vi "Send Command.vi"(7 "VolatusAPI":refnum<class "VolatusAPI.lvclass">, 8 "error in (no error)":errorcluster, 10 "Value":bool, 11 "2WayValve in":refnum<class "2WayValveH.lvclass">) -> (0 "error out":errorcluster, 3 "2WayValve out":refnum<class "2WayValveH.lvclass">)   [LabVIEW 2020, in "VolatusGUIElements.lvlib" / "2WayValveH.lvclass"]
uses:
  2WayValveH.lvclass
  Volatus/VolatusAPI/VolatusAPI.lvclass
  2WayValveH.lvclass/2WayValveH.ctl
  messages/CmdDigital/Class/Msg.lvclass/Msg.ctl
  Volatus/VolatusAPI/VolatusAPI.lvclass/VolatusAPI.ctl
  messages/CmdDigital/Class/Msg.lvclass
  C:/dev/lv20CE/relink/lv-protoc/LV-Proto/Message/Message.lvclass
  lv-vecto/Vecto/TCPMessageService/Send Message.vi
  <vilib>/Utility/error.llb/Error Cluster From Error Code.vi
  lv-protoc/LV-Proto/Message/Message.lvclass
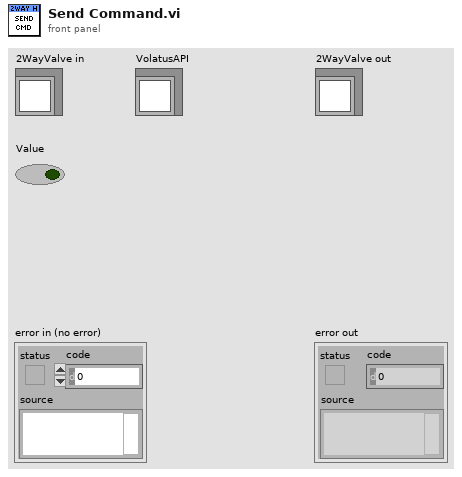
[diagram p1: front panel]
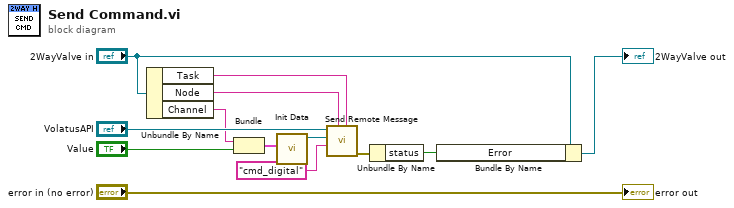
[diagram p0: block diagram]
diagram:
  n1 = Unbundle By Name("2WayValve in") -> ("Task"=w9:string, "Node"=w10:string, "Channel"=w8:string)
  n2 = Bundle("Channel"=w8, "Value"="Value") -> (w6:cluster{"Channel":string, "Value":bool})  [unwired: 1 in]
  n3 = call "Init Data.vi"("Data"=w6) -> ("Msg out"=w5:refnum<class "Msg.lvclass">)  [unwired: 10 in]
  n4 = call "Send Remote Message.vi"("Target Task (None)"=w9, "Target Node"=w10, "Message Type"="cmd_digital", "Message"=w5, "VolatusAPI in"="VolatusAPI") -> ("error out"=w2:errorcluster)  [unwired: 5 in, 1 out]
  n5 = Unbundle By Name(w2) -> ("status"=w1:bool)
  n6 = Bundle By Name(cluster="2WayValve in", "Error"=w1) -> (→"2WayValve out":refnum<class "2WayValveH.lvclass">)
  "error out" <- "error in (no error)"
